vi "Integrate channel from file.vi"(4 "Buffer size":i64=100000, 5 "Offset correction":dbl, 6 "Offset duration":dbl=0.0095, 7 "group name in":string="Untitled", 8 "Error In":errorcluster, 9 "Save data":bool, 10 "Integration settings":T1={"Channel"="CH0", "Output name"="Integral", "Factor"=-137722.0, "Start time"=0.0, "Duration"=3.0} {"Duration" format="%#_6p"; "Start time" format="%#_6p"}, 11 "File Path Control":path=path "\\\\eden\\NHMFLDATA/Data/Generator/December_2015/121715/rp163145_121715.tdms") -> (0 "Error Out":errorcluster, 1 "Integrated Waveform":waveform(dbl), 2 "Min max":cluster{"Max":dbl, "Min":dbl}, 3 "File Path out":path)   [LabVIEW 2015]
uses:
  Utilities/Controls/Integrate channel.ctl
  <vilib>/Waveform/WDTOps.llb/WDT Number of Waveform Samples DBL.vi
  <vilib>/Waveform/WDTOps.llb/WDT Append Waveforms DBL.vi
panel:
  out "Waveform Graph":waveform(dbl)(graph)
  # "Input CH            Factor              Output CH      Start              Duration"
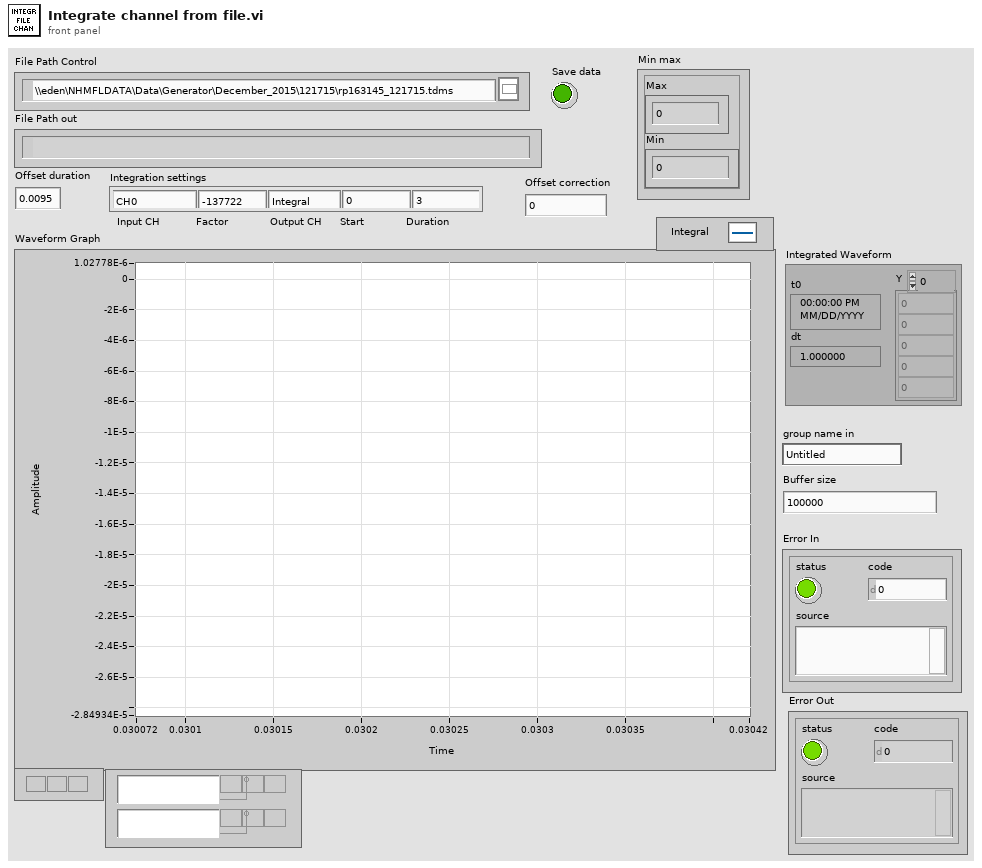
[diagram p1: front panel]
types:
  T1 = typedef "Integrate channel.ctl" = cluster{"Channel":string, "Output name":string, "Factor":dbl, "Start time":dbl, "Duration":dbl}
  T2 = enum16{"open", "open or create", "create or replace", "create", "open (read-only)"}
  T3 = typedef "TDMS channel info.ctl" = cluster{"t0":timestamp, "dt":dbl, "Channel length":i64}
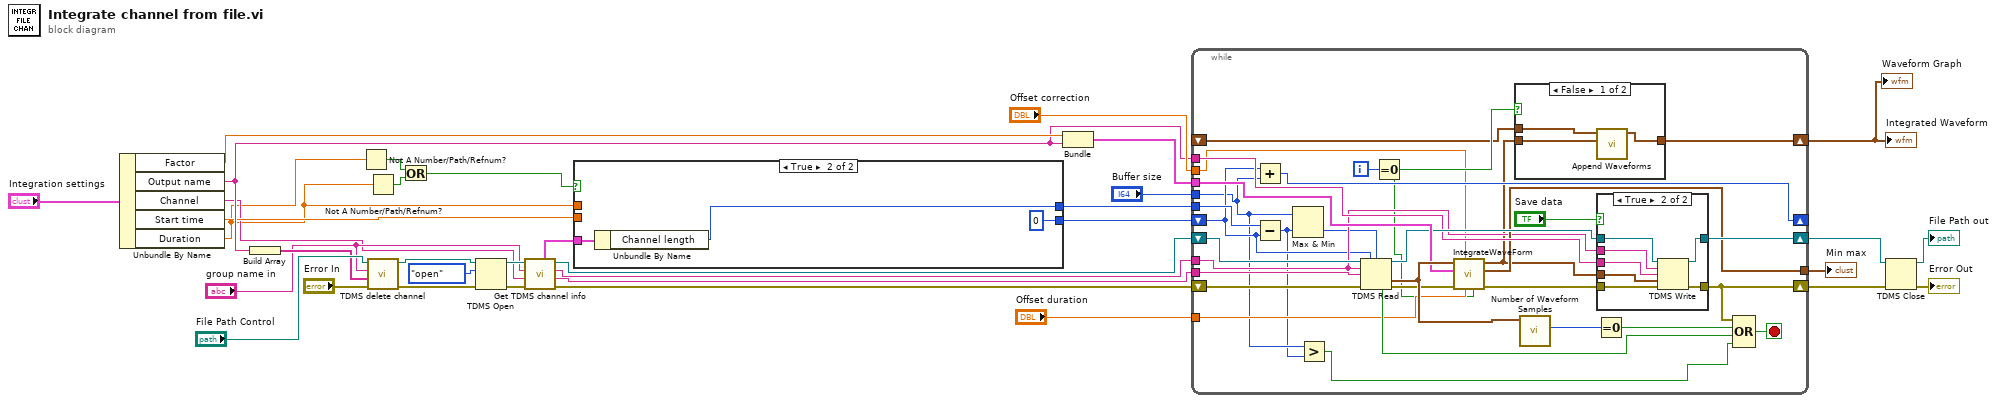
[diagram p0: block diagram]
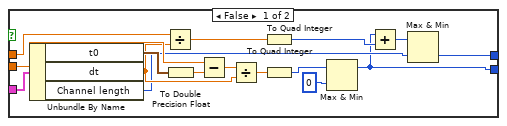
[diagram p2: hidden frame]
diagram:
  n1 = Unbundle By Name("Integration settings") -> ("Factor"=w33:dbl, "Output name"=w19:string, "Channel"=w12:string, "Start time"=w17:dbl, "Duration"=w4:dbl)
  n2 = Build Array(w19) -> (w18:string[])
  n3 = Not A Number/Path/Refnum?(number/path/refnum=w4) -> (NaN/Path/Refnum?=w3:bool)
  n4 = Not A Number/Path/Refnum?(number/path/refnum=w4) -> (NaN/Path/Refnum?=w2:bool)
  n5 = call "TDMS delete channel.vi"("error in (no error)"="Error In", "Channels"=w18, "group name"="group name in", "file path"="File Path Control") -> ("error out"=w20:errorcluster, "file path out"=w22:path)  [unwired: 5 in, 1 out]
  n6 = Or(x=w3, y=w2) -> (x .or. y?=w1:bool)
  n7 = TDMS Open(8:w20, 10:T2."open" ("operation (0:open)"), 11:w22) -> (0:w15:errorcluster, 3:w14:refnum<k34>)  [unwired: 4 in]
  n8 = call "Get TDMS channel info.vi"("error in"=w15, "Channel name"=w12, "group name"="group name in", "tdms file"=w14) -> ("error out"=w8:errorcluster, "channel name out"=w10:string, "group name out"=w11:string, "tdms file out"=w9:refnum<k34>, "TDMS channel info"=w7:T3)  [unwired: 3 in]
  n9 = case shown="True" w1 {
    tunnel: w17 -> [w49 _]
    tunnel: w4 -> [w48 _]
    tunnel: [w36 i64 0] -> w16
    tunnel: w7 -> [w44 w53]
    tunnel: [w39 w52] -> w6
    frame False {
      n10 = Unbundle By Name(w44) -> ("t0"=w51:timestamp, "dt"=w47:dbl, "Channel length"=w41:i64)
      n11 = Divide(x=w48, y=w47) -> (x/y=w40:dbl)
      n12 = To Double Precision Float(number=w51) -> (double precision float=w50:dbl)
      n13 = Subtract(x=w49, y=w50) -> (x-y=w43:dbl)
      n14 = Divide(x=w43, y=w47) -> (x/y=w46:dbl)
      n15 = To Quad Integer(1:w40) -> (0:w37:i64)
      n16 = To Quad Integer(1:w46) -> (0:w45:i64)
      n17 = Max & Min(x=w45, y=i64 0) -> (max(x,y)=w36:i64)  [unwired: 1 out]
      n18 = Add(x=w36, y=w37) -> (x+y=w38:i64)
      n19 = Max & Min(x=w38, y=w41) -> (min(x,y)=w39:i64)  [unwired: 1 out]
    }
    frame True {
      n20 = Unbundle By Name(w53) -> ("Channel length"=w52:i64)
    }
  }
  n21 = Bundle("Factor"=w33, "Output name"=w19) -> (w32:cluster{"Factor":dbl, "Output name":string})  [unwired: 1 in]
  n22 = while {
    tunnel: w10 -> [w84]
    tunnel: w32 -> [w82]
    tunnel: w19 -> [w80]
    shift-right: [w73] -> w31
    shift-left: w8 -> [w76]
    shift-right: [w74] -> w29
    shift-left: w9 -> [w86]
    tunnel: "Buffer size" -> [w57]
    shift-right: [w71] -> _
    shift-left: w16 -> [w59]
    tunnel: "Offset duration" -> [w69]
    tunnel: [w68] -> w25
    tunnel: w11 -> [w67]
    shift-right: [w64] -> w5
    shift-left: _ -> [w62]
    tunnel: "Offset correction" -> [w61]
    tunnel: w6 -> [w60]
    i -> [w70]
    stop <- w75 stop-if-true
    n23 = Add(x=w59, y=w57) -> (x+y=w71:i64)
    n24 = Subtract(x=w60, y=w59) -> (x-y=w56:i64)
    n25 = Max & Min(x=w57, y=w56) -> (min(x,y)=w58:i64)  [unwired: 1 out]
    n26 = Greater?(x=w57, y=w56) -> (0:w55:bool)
    n27 = TDMS Read(0:w86, 1:w59, 2:w58, 5:w67, 7:w84, 11:w76) -> (4:w81:refnum<k34>, 10:w83:waveform(dbl), 14:w72:bool, 15:w79:errorcluster)  [unwired: 2 in, 2 out]
    n28 = Equal To 0?(x=w70) -> (x = 0?=w65:bool)
    n29 = call "IntegrateWaveForm.vi"("First chunk?"=w65, "Offset duration"=w69, "Offset correction"=w61, "error in (no error)"=w79, "Integrate settings"=w82, "Waveform"=w83) -> ("error out"=w78:errorcluster, "Min max"=w68:cluster{"Max":dbl, "Min":dbl}, "Integrated Waveform"=w63:waveform(dbl))  [unwired: 3 in]
    n30 = case shown="False" w65 {
      tunnel: [w87 w90] -> w64
      tunnel: w63 -> [w88 w90]
      tunnel: w62 -> [w89 _]
      frame False {
        n31 = call-poly <vilib>:"Append Waveforms.vi"("waveform B"=w88, "waveform A"=w89) -> ("waveform out"=w87:waveform(dbl))  [unwired: 8 in, 1 out]
      }
      frame True {
      }
    }
    n32 = call-poly <vilib>:"Number of Waveform Samples.vi"("waveform in"=w83) -> ("number of samples"=w85:i32)  [unwired: 8 in, 2 out]
    n33 = Equal To 0?(x=w85) -> (x = 0?=w77:bool)
    n34 = case shown="True" "Save data" {
      tunnel: w81 -> [w92 w99]
      tunnel: w80 -> [_ w98]
      tunnel: w63 -> [_ w97]
      tunnel: w78 -> [w91 w96]
      tunnel: [w92 w95] -> w74
      tunnel: [w91 w94] -> w73
      tunnel: w67 -> [_ w93]
      frame False {
      }
      frame True {
        n35 = TDMS Write(0:w99, 5:w93, 7:w98, 9:w97, 11:w96) -> (4:w95:refnum<k34>, 15:w94:errorcluster)  [unwired: 1 in, 2 out]
      }
    }
    n36 = Compound Arithmetic op=OR(w73, w77, w72, w55) -> (w75:bool)
  }
  "Min max" <- w25
  "Integrated Waveform" <- w5
  "Waveform Graph" <- w5
  n37 = TDMS Close(8:w31, 11:w29) -> (0:→"Error Out":errorcluster, 3:→"File Path out":path)
